vi "Insert Trial Timestamp to Db.vi"(8 "error in (no error)":errorcluster, 10 "Timetsamp Time":timestamp, 11 "TrialBasedExperiment in":refnum<class "TrialBasedExperiment.lvclass">) -> (0 "error out":errorcluster, 3 "TrialBasedExperiment out":refnum<class "TrialBasedExperiment.lvclass">)   [LabVIEW 2012, in "AcquisitionCoreObjects.lvlib" / "TrialBasedExperiment.lvclass"]
uses:
  TrialBasedExperiment.lvclass
  <vilib>/addons/database/NI_Database_API.lvlib
  Acquisition/AcquistionObject/AcquistionObject.lvclass
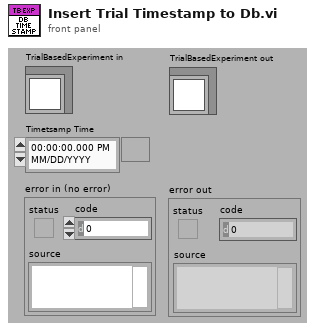
[diagram p1: front panel]
types:
  T1 = cluster{"setup":u8, "subject_id":i32, "session_start_time":dbl, "stim_start_time":dbl, "time":dbl}
  T2 = typedef "NI_Database_API.lvlib/Conn ObjectReference.ctl" = refnum<k1>
  T3 = typedef "StimulationPrimary.ctl" = cluster{"setup":u8, "subject_id":i32, "session_start_time":dbl, "stim_start_time":dbl}
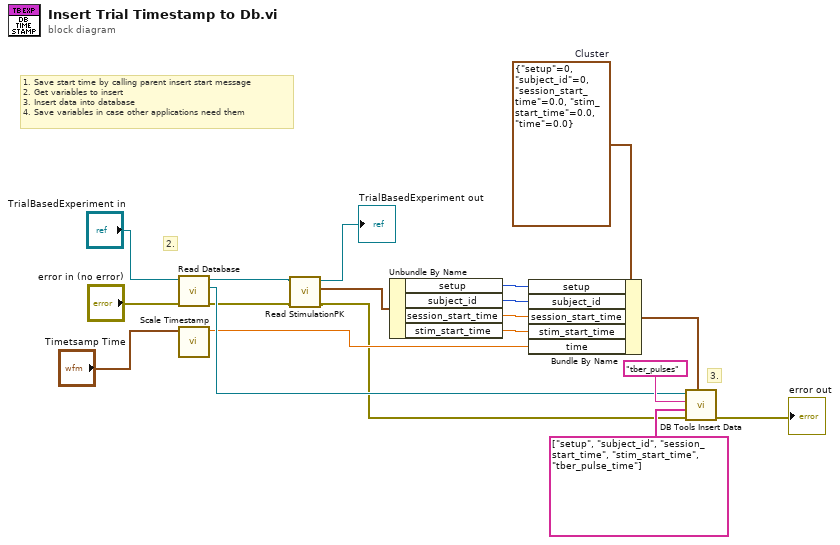
[diagram p0: block diagram]
diagram:
  w19 = T1 {"setup"=0, "subject_id"=0, "session_start_time"=0.0, "stim_start_time"=0.0, "time"=0.0}  # Cluster
  # "2."
  # "3."
  # "1. Save start time by calling parent insert start message\n2. Get variables to insert\n3. Insert data into database\n4. Save variables in case other applications need them"
  n1 = call-dynamic "Read Database.vi"("error in (no error)"="error in (no error)", "AcquistionObject in"="TrialBasedExperiment in") -> ("error out"=w5:errorcluster, "reference"=w13:T2, "AcquistionObject out"=w4:refnum<class "TrialBasedExperiment.lvclass">)  [unwired: 7 in]
  n2 = call "Scale Timestamp.vi"("Time Stamp"="Timetsamp Time") -> ("Scaled timestamp"=w9:dbl)  [unwired: 10 in]
  n3 = call-dynamic "Read StimulationPK.vi"("error in (no error)"=w5, "TrialBasedExperiment in"=w4) -> ("error out"=w2:errorcluster, "StimulationPK"=w3:T3, "TrialBasedExperiment out"=→"TrialBasedExperiment out":refnum<class "TrialBasedExperiment.lvclass">)  [unwired: 7 in]
  n4 = Unbundle By Name(w3) -> ("setup"=w16:u8, "subject_id"=w15:i32, "session_start_time"=w6:dbl, "stim_start_time"=w12:dbl)
  n5 = Bundle By Name(cluster=w19, "setup"=w16, "subject_id"=w15, "session_start_time"=w6, "stim_start_time"=w12, "time"=w9) -> (w14:T1)
  n6 = call <vilib>:"DB Tools Insert Data.vi"("data"=w14, "error in (no error)"=w2, "columns"=string[] ["setup", "subject_id", "session_start_time", "stim_start_time", "tber_pulse_time"], "table"="tber_pulses", "connection reference"=w13) -> ("error out"=→"error out":errorcluster)  [unwired: 5 in, 1 out]
